vi "Get Token.vi"(8 "error in (no error)":errorcluster, 11 "Event in":refnum<class "Event.lvclass">) -> (0 "error out":errorcluster, 2 "EventToken":refnum<class "EventToken.lvclass">, 3 "Event out":refnum<class "Event.lvclass">)   [LabVIEW 2009, in "EventManagerLibrary.lvlib" / "Event.lvclass"]
uses:
  Event.lvclass
  EventToken/EventToken.lvclass
  Event.lvclass/Event.ctl
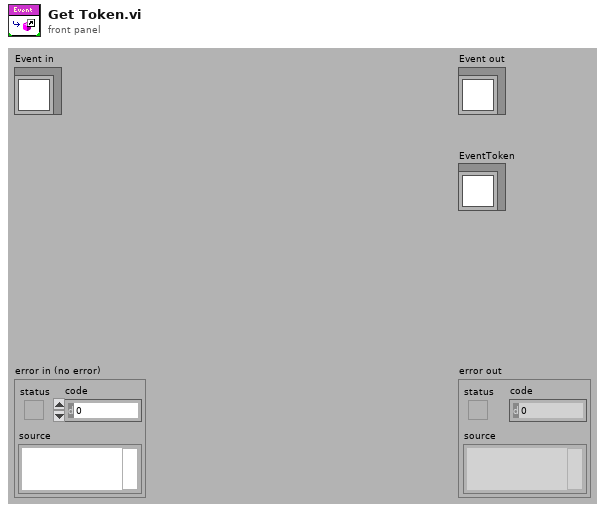
[diagram p1: front panel]
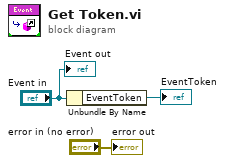
[diagram p0: block diagram]
diagram:
  n1 = Unbundle By Name("Event in") -> ("EventToken"=→"EventToken":refnum<class "EventToken.lvclass">)
  "error out" <- "error in (no error)"
  "Event out" <- "Event in"
